vi "Measure DAQ Voltages.vi"(8 "error in (no error)":errorcluster, 10 "Descriptions":string[](array[string]), 11 "Array in":refnum<k24>[](array[refnum])) -> (2 "Raw Voltages":dbl[](array[numeric]), 3 "Array out":refnum<k24>[](array[refnum]), 5 "Sensor Cluster":T1)   [LabVIEW 2016]
uses:
  C:/Program Files (x86)/National Instruments/LabVIEW 2016/vi.lib/ULx/ULx_LV.dll
  controls/MCC DAQ Readings.ctl
  <vilib>/ULx/Read.llb/ULx Read (Analog DBL 1Chan 1Samp).vi
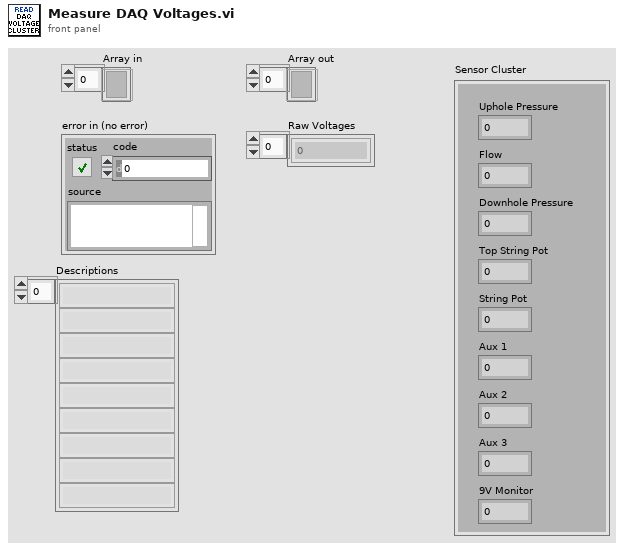
[diagram p1: front panel]
types:
  T1 = typedef "MCC DAQ Readings.ctl" = cluster{"Uphole Pressure":dbl, "Flow":dbl, "Downhole Pressure":dbl, "Top String Pot":dbl, "String Pot":dbl, "Aux 1":dbl, "Aux 2":dbl, "Aux 3":dbl, "9V Monitor":dbl}
  T2 = cluster{"[0]":dbl, "[1]":dbl, "[2]":dbl, "[3]":dbl, "[4]":dbl, "[5]":dbl, "[6]":dbl, "[7]":dbl, "[8]":dbl}
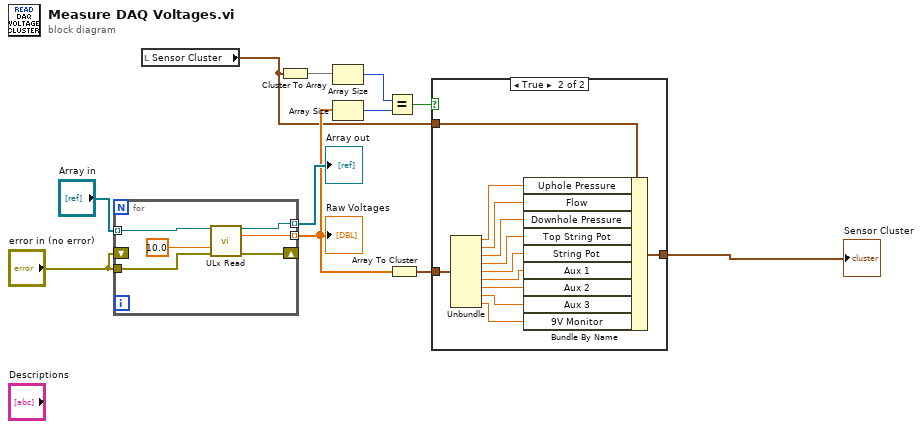
[diagram p0: block diagram]
diagram:
  n1 = for {
    tunnel: "Array in" -> [w17] mode=indexing
    tunnel: "error in (no error)" -> [w16]
    tunnel: [w14] -> w10 mode=indexing
    tunnel: [w12] -> w4 mode=indexing
    shift-right: [w13] -> _
    shift-left: "error in (no error)" -> [_]
    n2 = call-poly <vilib>:"ULx Read.vi"("task in"=w17, "timeout"=10.0, "error in"=w16) -> ("task out"=w14:refnum<k24>, "data"=w12:dbl, "error out"=w13:errorcluster)  [unwired: 10 in]
  }
  "Raw Voltages" <- w4
  "Array out" <- w10
  n3 = local read "Sensor Cluster"() -> (w1:T1)
  n4 = Cluster To Array(cluster=w1) -> (array=w8:dbl[])
  n5 = Array Size(array=w8) -> (size(s)=w6:i32)
  n6 = Array Size(array=w4) -> (size(s)=w5:i32)
  n7 = Equal?(x=w6, y=w5) -> (x = y?=w7:bool)
  n8 = Array To Cluster(array=w4) -> (cluster=w3:T2)
  n9 = case shown="True" w7 {
    tunnel: [w18 w30] -> w2
    tunnel: w1 -> [w18 w29]
    tunnel: w3 -> [_ w28]
    frame False {
    }
    frame True {
      n10 = Unbundle(w28) -> ("[0]"=w27:dbl, "[1]"=w26:dbl, "[2]"=w25:dbl, "[3]"=w24:dbl, "[4]"=w23:dbl, "[5]"=w22:dbl, "[6]"=w21:dbl, "[7]"=w20:dbl, "[8]"=w19:dbl)
      n11 = Bundle By Name(cluster=w29, "Uphole Pressure"=w27, "Flow"=w26, "Downhole Pressure"=w25, "Top String Pot"=w24, "String Pot"=w23, "Aux 1"=w22, "Aux 2"=w21, "Aux 3"=w20, "9V Monitor"=w19) -> (w30:T1)
    }
  }
  "Sensor Cluster" <- w2
